vi "PRUEBAS.vi"() -> ()   [LabVIEW 2025]
doc: "VI para hacer pruebas de funcionamiento de instrucciones y pines especificos\n(Este VI no deberia ser utilizable por estudiantes, solamente para pruebas, debugging o por docentes para explicar el funcionamiento de la trama de bytes)s"
panel:
  in  "stop":bool
  out "string":string
  out "error out":errorcluster
  out "return count":u32
  out "read buffer":string
  in  "VISA resource name":refnum<visa-resource-name>
  in  "Array":u8[](array[numeric]) format="%x"
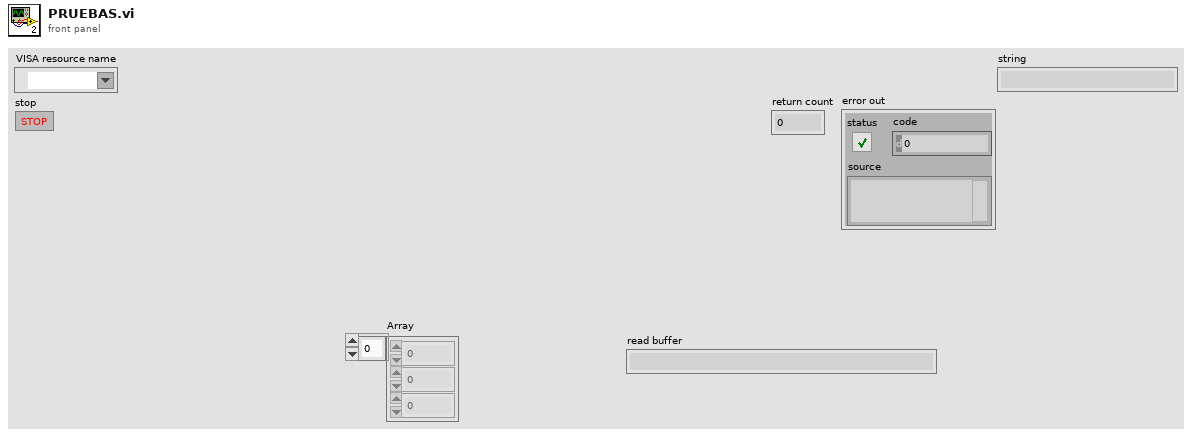
[diagram p1: front panel]
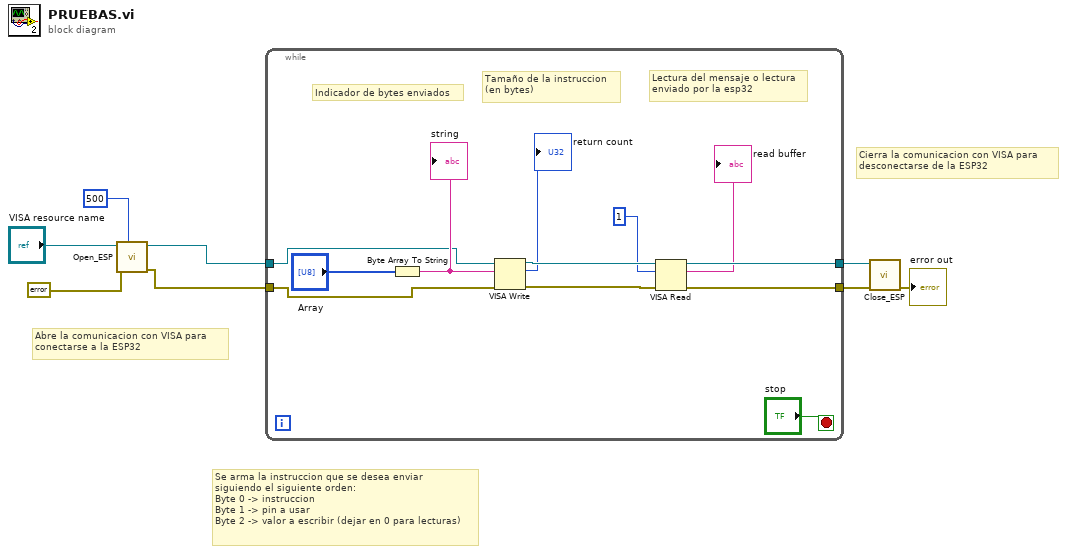
[diagram p0: block diagram]
diagram:
  # "Cierra la comunicacion con VISA para\ndesconectarse de la ESP32"
  # "Abre la comunicacion con VISA para\nconectarse a la ESP32"
  # "Se arma la instruccion que se desea enviar\nsiguiendo el siguiente orden:\nByte 0 -> instruccion\nByte 1 -> pin a usar\nByte 2 -> valor a escribir (dejar en 0 para lecturas)"
  n1 = call "Open_ESP.vi"("timeout (10sec)"=u32 500, "error in (no error)"=errorcluster {"status"=FALSE, "code"=0, "source"=""}, "VISA resource name"="VISA resource name") -> ("error out"=w4:errorcluster, "VISA resource name out"=w8:refnum<visa-resource-name>)  [unwired: 7 in]
  n2 = while {
    tunnel: w8 -> [w18]
    tunnel: [w14] -> w3
    tunnel: w4 -> [w17]
    tunnel: [w13] -> w2
    stop <- "stop" stop-if-true
    # "Lectura del mensaje o lectura\nenviado por la esp32"
    # "Tamaño de la instruccion\n(en bytes)"
    # "Indicador de bytes enviados"
    n3 = Byte Array To String(unsigned byte array="Array") -> (string=w19:string)
    "string" <- w19
    n4 = VISA Write(VISA resource name=w18, write buffer=w19, error in (no error)=w17) -> (VISA resource name out=w15:refnum<visa-resource-name>, return count=→"return count":u32, error out=w16:errorcluster)
    n5 = VISA Read(VISA resource name=w15, byte count=u32 1, error in (no error)=w16) -> (VISA resource name out=w14:refnum<visa-resource-name>, read buffer=→"read buffer":string, error out=w13:errorcluster)  [unwired: 1 out]
  }
  n6 = call "Close_ESP.vi"("error in (no error)"=w2, "VISA resource name"=w3) -> ("error out"=→"error out":errorcluster)  [unwired: 9 in]
